vi "check Sum2.vi"(10 "Array":dbl[](array[numeric])) -> (1 "subarray":i16[](array[numeric]))   [LabVIEW 2014]
panel:
  out "Numeric 2":i32
  out "Numeric":i32
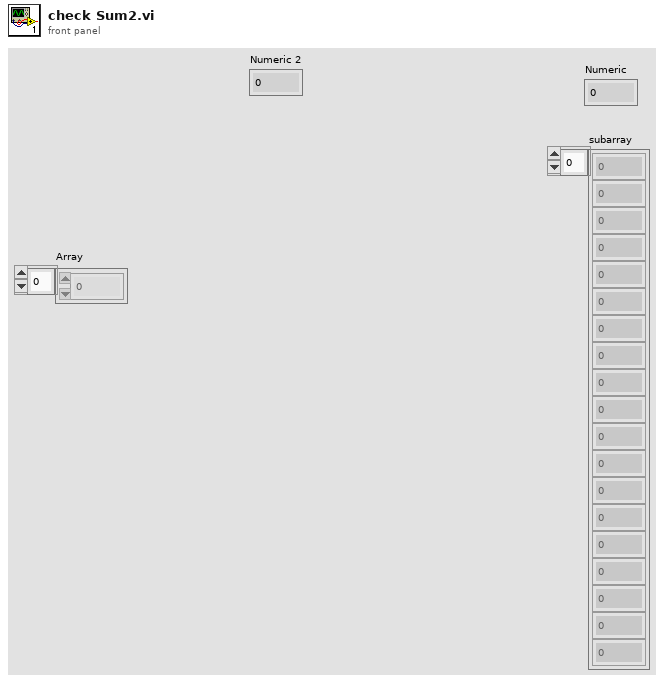
[diagram p1: front panel]
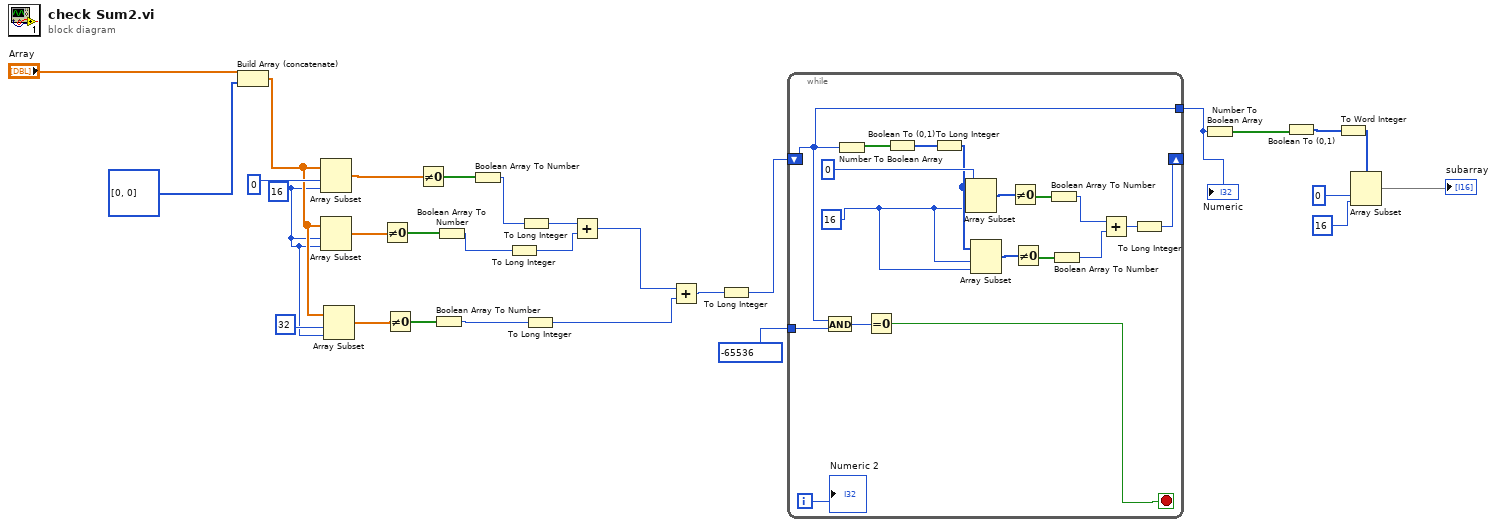
[diagram p0: block diagram]
diagram:
  w20 = 16
  n1 = Build Array (concatenate)("Array", i32[] [0, 0]) -> (w22:dbl[])
  n2 = Array Subset(array=w22, index=0, length=w20) -> (w26:dbl[])
  n3 = Array Subset(array=w22, index=w20, length=w20) -> (w23:dbl[])
  n4 = Array Subset(array=w22, index=32, length=w20) -> (w19:dbl[])
  n5 = Not Equal To 0?(x=w23) -> (x != 0?=w24:bool[])
  n6 = Not Equal To 0?(x=w19) -> (x != 0?=w18:bool[])
  n7 = Not Equal To 0?(x=w26) -> (x != 0?=w25:bool[])
  n8 = Boolean Array To Number(Boolean array=w18) -> (number=w3:u32)
  n9 = Boolean Array To Number(Boolean array=w24) -> (number=w5:u32)
  n10 = Boolean Array To Number(Boolean array=w25) -> (number=w6:u32)
  n11 = To Long Integer(number=w5) -> (32bit integer=w4:i32)
  n12 = To Long Integer(number=w6) -> (32bit integer=w7:i32)
  n13 = To Long Integer(number=w3) -> (32bit integer=w2:i32)
  n14 = Add(x=w7, y=w4) -> (x+y=w16:i32)
  n15 = Add(x=w16, y=w2) -> (x+y=w15:i32)
  n16 = To Long Integer(number=w15) -> (32bit integer=w14:i32)
  n17 = while {
    tunnel: -65536 -> [w47]
    shift-right: [w32] -> _
    shift-left: w14 -> [w31]
    tunnel: [w31] -> w1
    i -> [w30]
    stop <- w45 stop-if-true
    w40 = 16
    n18 = And(x=w31, y=w47) -> (x .and. y?=w46:i32)
    n19 = Number To Boolean Array(number=w31) -> (Boolean array=w43:bool[])
    n20 = Equal To 0?(x=w46) -> (x = 0?=w45:bool)
    n21 = Boolean To (0,1)(Boolean=w43) -> (0, 1=w42:i16[])
    n22 = To Long Integer(number=w42) -> (32bit integer=w41:i32[])
    n23 = Array Subset(array=w41, index=0, length=w40) -> (w39:i32[])
    n24 = Array Subset(array=w41, index=w40, length=w40) -> (w36:i32[])
    n25 = Not Equal To 0?(x=w39) -> (x != 0?=w38:bool[])
    n26 = Not Equal To 0?(x=w36) -> (x != 0?=w37:bool[])
    n27 = Boolean Array To Number(Boolean array=w38) -> (number=w35:u32)
    n28 = Boolean Array To Number(Boolean array=w37) -> (number=w34:u32)
    n29 = Add(x=w35, y=w34) -> (x+y=w33:u32)
    n30 = To Long Integer(number=w33) -> (32bit integer=w32:i32)
    "Numeric 2" <- w30
  }
  "Numeric" <- w1
  n31 = Number To Boolean Array(number=w1) -> (Boolean array=w8:bool[])
  n32 = Boolean To (0,1)(Boolean=w8) -> (0, 1=w11:i16[])
  n33 = To Word Integer(number=w11) -> (16bit integer=w10:i16[])
  n34 = Array Subset(array=w10, index=0, length=16) -> (→"subarray":i16[])
